vi "FlpLib DQtoAlphaBeta_noSine 4.vi"(0 "direct":sgl format="%#_30g", 1 "cosx":sgl, 2 "sinx":sgl, 5 "quadrature":sgl format="%#_30g") -> (4 "alpha":sgl format="%#_30g", 6 "beta":sgl format="%#_30g")   [LabVIEW 2017]
uses:
  <userlib>/_NI FLP Library/FPGA/outsideSCTL/FlpLib Multiply Shared Instance 4.vi
  <userlib>/_NI FLP Library/FPGA/outsideSCTL/FlpLib Add Shared Instance 4.vi
  <userlib>/_NI FLP Library/FPGA/outsideSCTL/FlpLib Subtract Shared Instance 4.vi
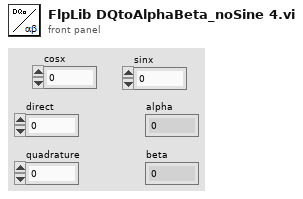
[diagram p1: front panel]
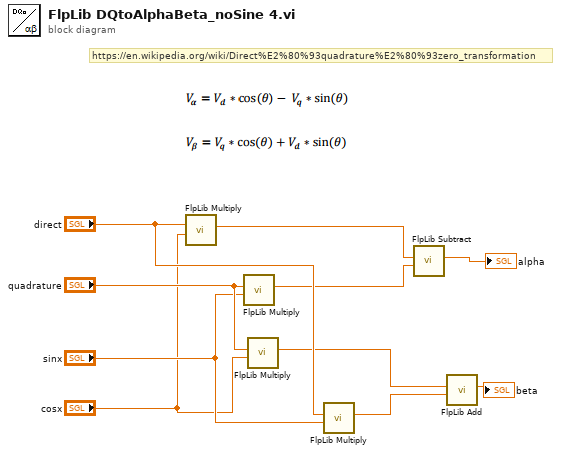
[diagram p0: block diagram]
diagram:
  # "https://en.wikipedia.org/wiki/Direct%E2%80%93quadrature%E2%80%93zero_transformation"
  n1 = call-poly <userlib>:"FlpLib Multiply.vi"("y"="cosx", "x"="direct") -> ("x*y"=w6:sgl)  [unwired: 5 in]
  n2 = call-poly <userlib>:"FlpLib Multiply.vi"("y"="sinx", "x"="quadrature") -> ("x*y"=w5:sgl)  [unwired: 5 in]
  n3 = call-poly <userlib>:"FlpLib Multiply.vi"("y"="cosx", "x"="quadrature") -> ("x*y"=w3:sgl)  [unwired: 5 in]
  n4 = call-poly <userlib>:"FlpLib Multiply.vi"("y"="sinx", "x"="direct") -> ("x*y"=w2:sgl)  [unwired: 5 in]
  n5 = call-poly <userlib>:"FlpLib Subtract.vi"("y"=w5, "x"=w6) -> ("x-y"=→"alpha":sgl)  [unwired: 5 in]
  n6 = call-poly <userlib>:"FlpLib Add.vi"("y"=w2, "x"=w3) -> ("x+y"=→"beta":sgl)  [unwired: 5 in]
